vi "Init.vi"() -> (3 "TEMPLATE Actor out":refnum<class "TEMPLATE Actor.lvclass">)   [LabVIEW 2020, in "_Template.lvlib" / "Templates.lvlib" / "TEMPLATE Actor.lvlib" / "TEMPLATE Actor.lvclass"]
uses:
  TEMPLATE Actor.lvclass
  jettl/jettl/Actor/Actor.lvlib
  C:/git/jettl/src/jettl Tools/_Template/Templates/TEMPLATE Actor/TEMPLATE Actor/TEMPLATE Actor.lvclass
  C:/git/jettl/src/jettl/jettl/Actor/Actor/Actor.lvclass
  C:/git/jettl/src/jettl/jettl/Decorator/Decorator.lvclass
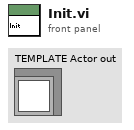
[diagram p1: front panel]
types:
  T1 = typedef "jettl.lvlib/Actor.lvlib/Msg Set.ctl" = set{refnum<class "Msg.lvclass">}
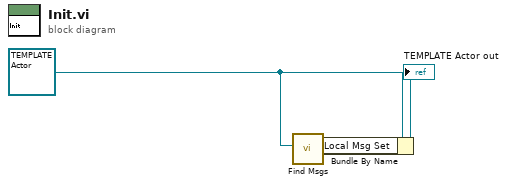
[diagram p0: block diagram]
diagram:
  w1 = refnum<class "TEMPLATE Actor.lvclass"> refnum ("TEMPLATE Actor out")
  n1 = call "Find Msgs.vi"("Actor"=w1) -> ("Msgs"=w2:T1)  [unwired: 10 in]
  n2 = Bundle By Name(cluster=w1, "Local Msg Set"=w2) -> (→"TEMPLATE Actor out":refnum<class "TEMPLATE Actor.lvclass">)
